vi "remove mappings to missing channels.vi"(8 "error in":errorcluster, 11 "Engine Parent Editor Node in":refnum<class "Engine Parent Editor Node.lvclass">) -> (0 "error out":errorcluster, 3 "Engine Parent Editor Node out":refnum<class "Engine Parent Editor Node.lvclass">)   [LabVIEW 2013, in "PL Framework Configuration Tool.lvlib" / "Engine Parent Editor Node.lvclass"]
uses:
  Engine Parent Editor Node.lvclass
  <vilib>/NI/Module Execution Interface/Engine Configuration/engine configuration.lvclass
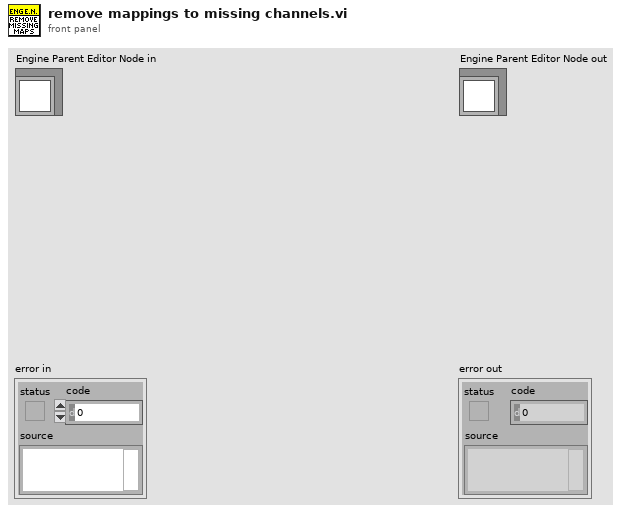
[diagram p1: front panel]
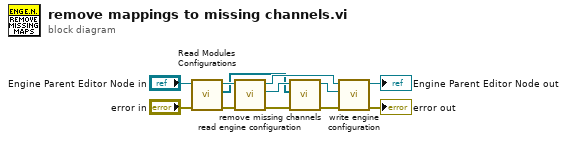
[diagram p0: block diagram]
diagram:
  n1 = call "Read Modules Configurations.vi"("error in"="error in", "Engine Parent in"="Engine Parent Editor Node in") -> ("error out"=w9:errorcluster, "Component Configurations"=w2:refnum<class "TBM module configuration.lvclass">[], "Engine Parent out"=w10:refnum<class "Engine Parent Editor Node.lvclass">)  [unwired: 7 in]
  n2 = call "read engine configuration.vi"("error in"=w9, "Engine Parent Editor Node in"=w10) -> ("error out"=w3:errorcluster, "engine configuration"=w8:refnum<class "engine configuration.lvclass">, "Engine Parent Editor Node out"=w7:refnum<class "Engine Parent Editor Node.lvclass">)  [unwired: 7 in]
  n3 = call <vilib>:"remove missing channels.vi"("error in"=w3, "module configurations"=w2, "engine configuration in"=w8) -> ("error out"=w4:errorcluster, "engine configuration out"=w5:refnum<class "engine configuration.lvclass">)  [unwired: 7 in]
  n4 = call "write engine configuration.vi"("error in"=w4, "engine configuration"=w5, "Engine Parent Editor Node in"=w7) -> ("error out"=→"error out":errorcluster, "Engine Parent Editor Node out"=→"Engine Parent Editor Node out":refnum<class "Engine Parent Editor Node.lvclass">)  [unwired: 7 in]
